vi "String - Check BOM B4 Convert to Unicode String.vi"(11 "Check 0xFFEE":string) -> (3 "Convert ASCII to Unicode":string)   [LabVIEW 2013]
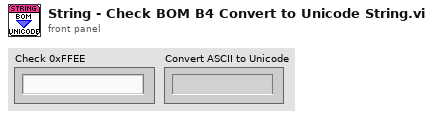
[diagram p1: front panel]
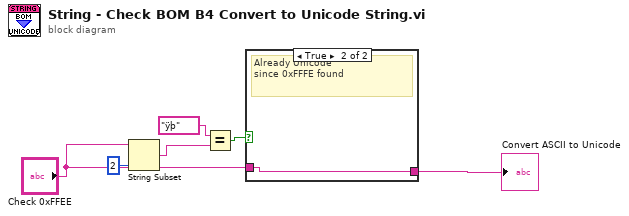
[diagram p0: block diagram]
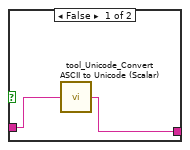
[diagram p2: hidden frame]
diagram:
  n1 = String Subset(string="Check 0xFFEE", length (rest)=2 ("length (rest)")) -> (substring=w4:string)  [unwired: 1 in]
  n2 = Equal?(x="ÿþ" ("y"), y=w4) -> (x = y?=w6:bool)
  n3 = case shown="True" w6 {
    tunnel: "Check 0xFFEE" -> [w8 w9]
    tunnel: [w7 w9] -> w2
    frame False {
      n4 = call "tool_Unicode_Convert ASCII to Unicode (Scalar).vi"("ASCII"=w8) -> ("Unicode"=w7:string)  [unwired: 4 in]
    }
    frame True {
      # "Already Unicode\nsince 0xFFFE found"
    }
  }
  "Convert ASCII to Unicode" <- w2
